vi "Byte Buffer.Read (I16).vi"(8 "error in (no error)":errorcluster, 10 "buffer offset":u64, 11 "Byte Buffer in":refnum<class "Byte Buffer.lvclass">) -> (0 "error out":errorcluster, 1 "value":i16, 2 "new buffer offset":u64, 3 "Byte Buffer out":refnum<class "Byte Buffer.lvclass">)   [LabVIEW 2016, in "VeriStand Data.lvlib" / "Byte Buffer.lvclass"]
doc: "Reads one element of data from the provided <B>Byte Buffer</B> at location <B>buffer offset</B> in the format of the data type specified."
uses:
  Byte Buffer.lvclass
  Byte Buffer.lvclass/Byte Buffer.ctl
  Byte Buffer.Read.Typed String.vi
  Byte Buffer.Subset.Get.vi
  Utilities/Utilities.Sizeof.Array.vi
  Utilities/Utilities.Buffer.String.vi
  Byte Buffer.Get Buffer Size.vi
  Memory Management/Memory Management.MoveByteBlock.Write (String).vi
  Byte Buffer.Get Buffer Pointer.vi
  Utilities/Utilities.Sizeof.Scalar.vi
  Byte Buffer.Get Byte Order.vi
  Memory Management/Memory Management.Handle Return.vi
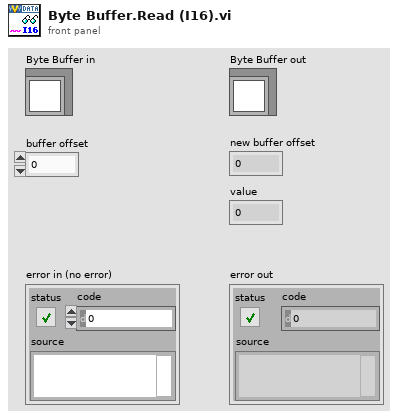
[diagram p1: front panel]
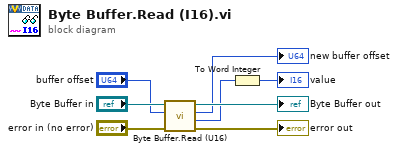
[diagram p0: block diagram]
diagram:
  n1 = call "Byte Buffer.Read (U16).vi"("error in (no error)"="error in (no error)", "buffer offset"="buffer offset", "Byte Buffer in"="Byte Buffer in") -> ("error out"=→"error out":errorcluster, "value"=w3:u16, "new buffer offset"=→"new buffer offset":u64, "Byte Buffer out"=→"Byte Buffer out":refnum<class "Byte Buffer.lvclass">)  [unwired: 5 in]
  n2 = To Word Integer(number=w3) -> (16bit integer=→"value":i16)
